vi "Untitled 9.vi"() -> ()   [LabVIEW 2013]
panel:
  in  "Tab Control":T1(tab)
  in  "Numeric":dbl=33.3
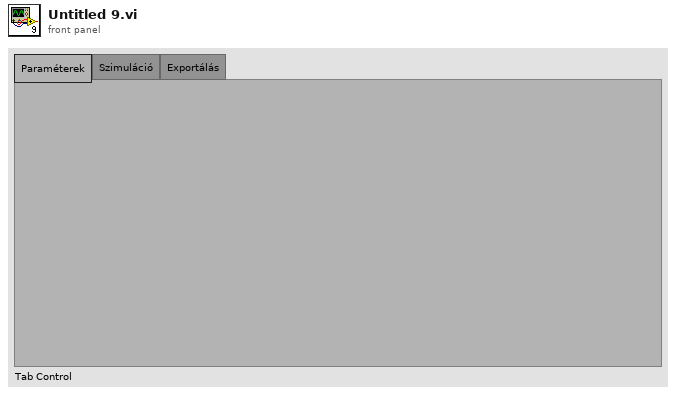
[diagram p1: front panel]
types:
  T1 = enum32{"Paraméterek", "Szimuláció", "Exportálás"}
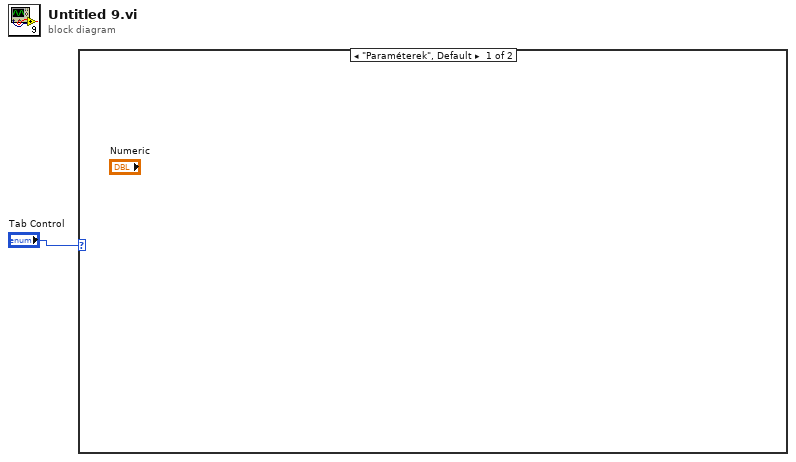
[diagram p0: block diagram]
diagram:
  n1 = case shown="\"Paraméterek\", Default" "Tab Control" {
    frame "Paraméterek", Default {
    }
    frame "Szimuláció" {
    }
  }
